vi "关键参数交互.vi"() -> ()   [LabVIEW 2016, in "CODCr库.lvlib"]
panel:
  out "x != y?":T1
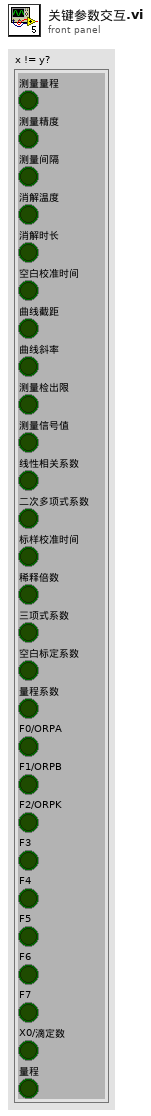
[diagram p1: front panel]
types:
  T1 = cluster{"测量量程":bool, "测量精度":bool, "测量间隔":bool, "消解温度":bool, "消解时长":bool, "空白校准时间":bool, "曲线截距":bool, "曲线斜率":bool, "测量检出限":bool, "测量信号值":bool, "线性相关系数":bool, "二次多项式系数":bool, "标样校准时间":bool, "稀释倍数":bool, "三项式系数":bool, "空白标定系数":bool, "量程系数":bool, "F0/ORPA":bool, "F1/ORPB":bool, "F2/ORPK":bool, "F3":bool, "F4":bool, "F5":bool, "F6":bool, "F7":bool, "X0/滴定数":bool, "量程":bool}
  T2 = cluster{"chose":string, "公式":cluster{"X^2":dbl, "X":dbl, "b":dbl}}
  T3 = cluster{"测量量程":dbl, "测量精度":dbl, "测量间隔":dbl, "消解温度":dbl, "消解时长":dbl, "空白校准时间":timestamp, "曲线截距":dbl, "曲线斜率":dbl, "测量检出限":dbl, "测量信号值":dbl, "线性相关系数":dbl, "二次多项式系数":dbl, "标样校准时间":timestamp, "稀释倍数":dbl, "三项式系数":dbl, "空白标定系数":dbl, "量程系数":dbl, "F0/ORPA":dbl, "F1/ORPB":dbl, "F2/ORPK":dbl, "F3":dbl, "F4":dbl, "F5":dbl, "F6":dbl, "F7":dbl, "X0/滴定数":dbl, "量程":dbl}
  T4 = cluster{"时间标识":timestamp, "设备":string, "日志信息":string, "流程参数":string}
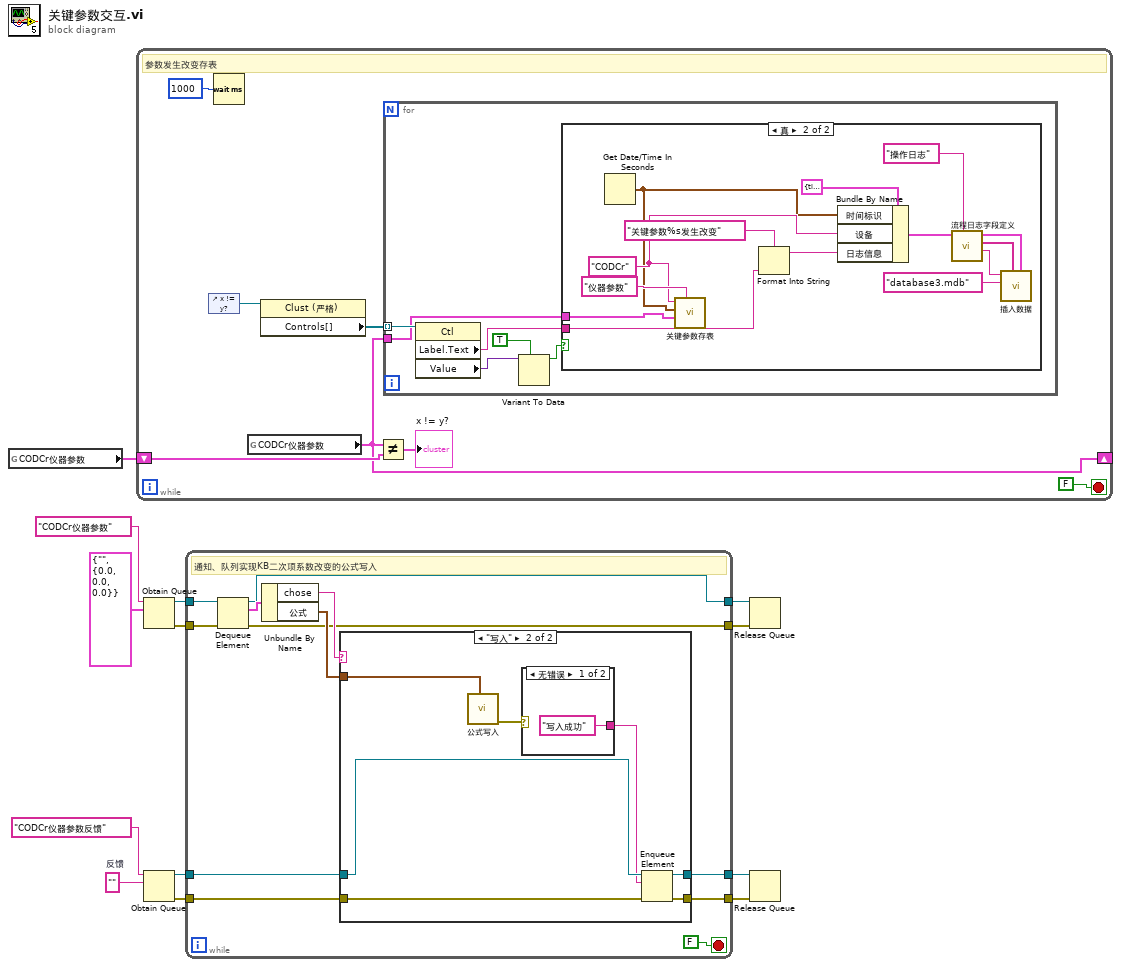
[diagram p0: block diagram]
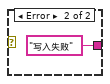
[diagram p3: hidden frame]
diagram:
  w4 = ""  # 反馈
  n1 = global read "CODcr全局变量.vi" "CODCr仪器参数"() -> (w13:T3)
  n2 = while {
    shift-right: [w14] -> _
    shift-left: w13 -> [w18]
    stop <- FALSE stop-if-true
    # "参数发生改变存表"
    n3 = control-ref of="x != y?"() -> (w16:refnum<vi>)
    n4 = Wait (ms)(milliseconds to wait=u32 1000 ("等待时间（毫秒）")) -> ()  [unwired: 1 out]
    n5 = global read "CODcr全局变量.vi" "CODCr仪器参数"() -> (w14:T3)
    n6 = property class="Clust (严格)"(reference=w16) -> ("Controls[]"=w15:refnum<vi>[])  [unwired: 1 in, 2 out]
    n7 = Not Equal?(x=w14, y=w18) -> (x != y?=→"x != y?":T1)
    n8 = for {
      tunnel: w15 -> [w26] mode=indexing
      tunnel: w14 -> [w22]
      n9 = property class="Ctl"(reference=w26) -> ("Label.Text"=w21:string, "Value"=w25:variant)  [unwired: 1 in, 2 out]
      n10 = Variant To Data(type=TRUE, Variant=w25) -> (data=w23:bool)  [unwired: 1 in, 1 out]
      n11 = case shown="真" w23 {
        tunnel: w22 -> [_ w27]
        tunnel: w21 -> [_ w38]
        frame False {
        }
        frame True {
          w29 = "CODCr" ("仪器名称")
          n12 = Get Date/Time In Seconds() -> (seconds since 1Jan1904=w28:timestamp)
          n13 = call "关键参数存表.vi"("table"="仪器参数", "仪器参数"=w27, "datatime"=w28, "仪器名称"=w29) -> ()  [unwired: 7 in, 1 out]
          n14 = Format Into String(format string="关键参数%s发生改变" ("格式字符串"), w38) -> (resulting string=w37:string)  [unwired: 2 in, 1 out]
          n15 = Bundle By Name(cluster=T4 {"时间标识"=timestamp(0 s since 1904-01-01), "设备"="", "日志信息"="", "流程参数"=""} ("data in"), "时间标识"=w28, "设备"=w29, "日志信息"=w37) -> (w31:T4)
          n16 = call "流程日志字段定义.vi"("table输入"="操作日志", "data in"=w31) -> ("table输出"=w34:string, "columns"=w35:string[], "data out"=w36:T4)  [unwired: 7 in]
          n17 = call "插入数据.vi"("data"=w36, "columns"=w35, "database"="database3.mdb", "table"=w34) -> ()  [unwired: 7 in, 1 out]
        }
      }
    }
  }
  n18 = Obtain Queue(name (unnamed)="CODCr仪器参数" ("名称（未命名）"), element data type=T2 {"chose"="", "公式"={"X^2"=0.0, "X"=0.0, "b"=0.0}}) -> (queue out=w12:refnum<queue>, error out=w11:errorcluster)  [unwired: 3 in, 1 out]
  n19 = Obtain Queue(name (unnamed)="CODCr仪器参数反馈" ("名称（未命名）"), element data type=w4) -> (queue out=w5:refnum<queue>, error out=w3:errorcluster)  [unwired: 3 in, 1 out]
  n20 = while {
    tunnel: w12 -> [w51]
    tunnel: w11 -> [w50]
    tunnel: [w46] -> w8
    tunnel: [w45] -> w7
    tunnel: w5 -> [w44]
    tunnel: w3 -> [w43]
    tunnel: [w42] -> w2
    tunnel: [w41] -> w1
    stop <- FALSE stop-if-true
    # "通知、队列实现KB二次项系数改变的公式写入"
    n21 = Dequeue Element(queue=w51, error in (no error)=w50) -> (queue out=w46:refnum<queue>, element=w49:T2, error out=w45:errorcluster)  [unwired: 1 in, 1 out]
    n22 = Unbundle By Name(w49) -> ("chose"=w48:string, "公式"=w47:cluster{"X^2":dbl, "X":dbl, "b":dbl})
    n23 = case shown="\"写入\"" w48 {
      tunnel: w47 -> [_ w56]
      tunnel: w44 -> [w54 w61]
      tunnel: w43 -> [w53 w59]
      tunnel: [w54 w58] -> w42
      tunnel: [w53 w57] -> w41
      frame "假", Default {
      }
      frame "写入" {
        n24 = call "公式写入.vi"("公式"=w56) -> ("error out"=w55:errorcluster)  [unwired: 10 in]
        n25 = case shown="无错误" w55 {
          tunnel: ["写入成功" ("消息") "写入失败" ("消息")] -> w60
          frame No Error {
          }
          frame Error {
          }
        }
        n26 = Enqueue Element(queue=w61, element=w60, error in (no error)=w59) -> (queue out=w58:refnum<queue>, error out=w57:errorcluster)  [unwired: 1 in, 1 out]
      }
    }
  }
  n27 = Release Queue(queue=w8, error in (no error)=w7) -> ()  [unwired: 1 in, 3 out]
  n28 = Release Queue(queue=w2, error in (no error)=w1) -> ()  [unwired: 1 in, 3 out]
